vi "set_detectors.vi"(8 "error in (no error)":errorcluster, 11 "DET_BUNCH in":refnum<class "Avantes_bunch.lvclass">) -> (0 "error out":errorcluster, 3 "DET_BUNCH out":refnum<class "Avantes_bunch.lvclass">)   [LabVIEW 2020, in "Avantes_bunch.lvclass"]
uses:
  Avantes_bunch.lvclass
  C:/Dev/TRANCON/Classes/GeneralFunctionality/GeneralFunctionality.lvclass
  GeneralFunctionality/GeneralFunctionality.lvclass/GeneralFunctionality.ctl
  Config/Config.lvclass
  UV-VIS_AVANTES/UV-VIS_AVANTES.lvclass
  C:/Dev/TRANCON/Classes/Detector/Detector.lvclass
  Config/Config.lvclass/Config.ctl
  UV-VIS_AVANTES/UV-VIS_AVANTES.lvclass/UV-VIS_AVANTES.ctl
  Avantes_bunch.lvclass/Avantes_bunch.ctl
  <userlib>/_OpenG.lib/dictionary/dictionary.llb/Dictionary Create__ogtk.vi
  <userlib>/_OpenG.lib/dictionary/dictionary.llb/Dictionary Update__ogtk.vi
  <userlib>/_OpenG.lib/dictionary/dictionary.llb/Dictionary Update (by scalar value)__ogtk.vi
  <userlib>/_OpenG.lib/dictionary/dictionary.llb/Dictionary Get Value__ogtk.vi
  GeneralFunctionality/GeneralFunctionality.lvclass
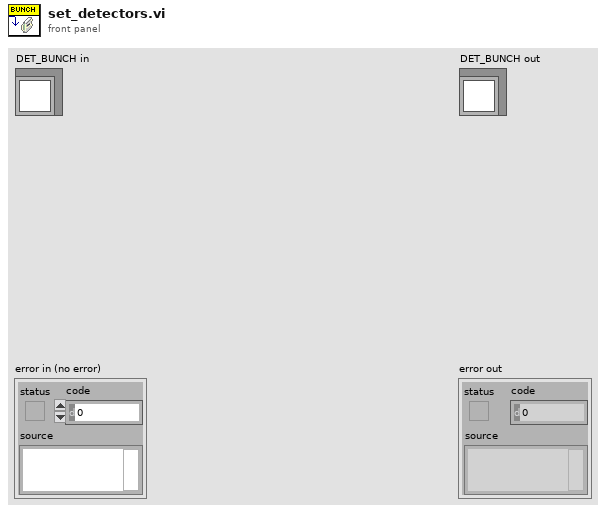
[diagram p1: front panel]
types:
  T1 = typedef "Rendezvous RefNum" = refnum<k1>
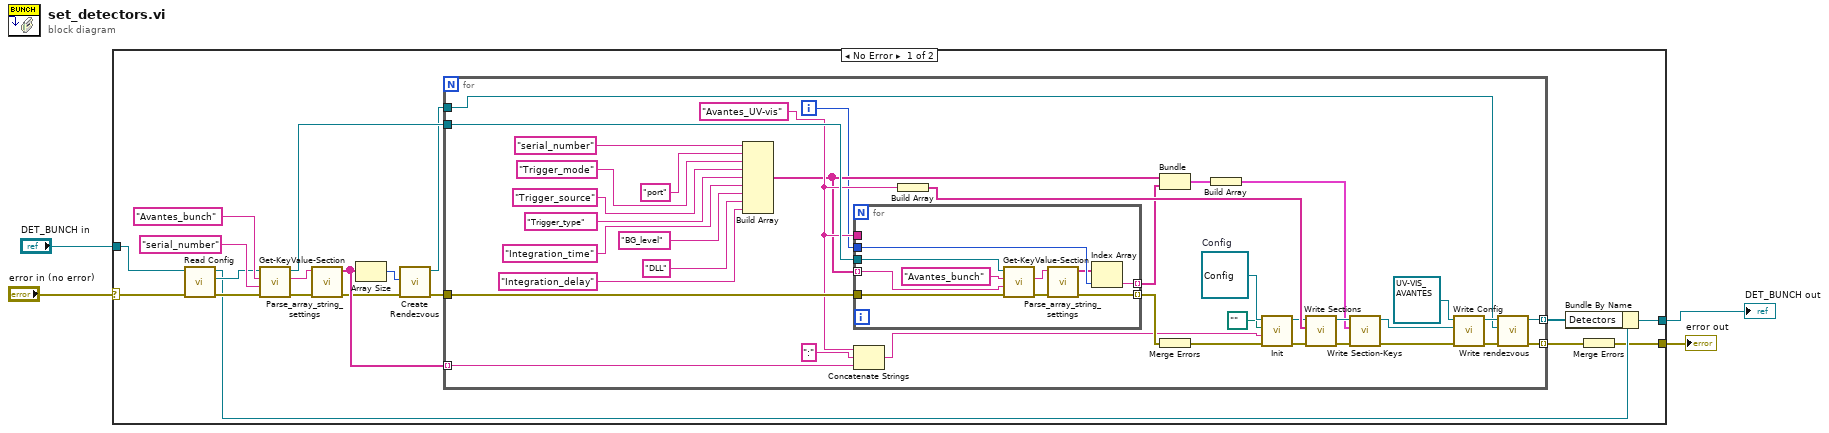
[diagram p0: block diagram]
diagram:
  n1 = case shown="No Error" "error in (no error)" {
    selector: "error in (no error)" -> [w15 w72]
    tunnel: [w11 w72] -> w3
    tunnel: [w10 w71] -> w1
    tunnel: "DET_BUNCH in" -> [w18 w71]
    frame No Error {
      n2 = call "Read Config.vi"("error in (no error)"=w15, "GeneralFunctionality en entrée"=w18) -> ("error out"=w16:errorcluster, "Config.lvclass"=w17:refnum<class "Config.lvclass">, "GeneralFunctionality en sortie"=w14:refnum<class "Avantes_bunch.lvclass">)  [unwired: 7 in]
      n3 = call-dynamic "Get-KeyValue-Section.vi"("error in (no error)"=w16, "Key"="serial_number", "Section"="Avantes_bunch", "Config in"=w17) -> ("error out"=w22:errorcluster, "Value"=w21:string, "Config out"=w23:refnum<class "Config.lvclass">)  [unwired: 5 in]
      n4 = call "Parse_array_string_settings.vi"("error in (no error)"=w22, "Value"=w21) -> ("error out"=w7:errorcluster, "Output"=w9:string[])  [unwired: 8 in]
      n5 = Array Size(array=w9) -> (size(s)=w8:i32)
      n6 = call <vilib>:"Create Rendezvous.vi"("error in (no error)"=w7, "size (2)"=w8) -> ("error out"=w6:errorcluster, "rendezvous"=w5:T1)  [unwired: 3 in, 1 out]
      n7 = for {
        tunnel: w9 -> [w46] mode=indexing
        tunnel: w6 -> [w52]
        tunnel: [w25] -> w12 mode=indexing
        tunnel: w23 -> [w55]
        tunnel: [w26] -> w13 mode=indexing
        tunnel: w5 -> [w24]
        i -> [w34]
        w42 = "Avantes_UV-vis" ("Section")
        w50 = refnum<class "Config.lvclass"> refnum  # Config
        n8 = Build Array("serial_number" ("Key"), "port" ("Key"), "Trigger_mode" ("element"), "Trigger_source" ("element"), "Trigger_type" ("element"), "Integration_time" ("element"), "BG_level" ("element"), "DLL" ("element"), "Integration_delay" ("element")) -> (w40:string[])
        n9 = for {
          tunnel: w55 -> [w70]
          tunnel: w40 -> [w69] mode=indexing
          tunnel: w42 -> [_]
          tunnel: [w64] -> w41 mode=indexing
          tunnel: [w63] -> w51 mode=indexing
          tunnel: w52 -> [w68]
          tunnel: w34 -> [w65]
          n10 = call-dynamic "Get-KeyValue-Section.vi"("error in (no error)"=w68, "Key"=w69, "Section"="Avantes_bunch", "Config in"=w70) -> ("error out"=w62:errorcluster, "Value"=w66:string)  [unwired: 5 in, 1 out]
          n11 = call "Parse_array_string_settings.vi"("error in (no error)"=w62, "Value"=w66) -> ("error out"=w63:errorcluster, "Output"=w61:string[])  [unwired: 8 in]
          n12 = Index Array(array=w61, index=w65) -> (element=w64:string)
        }
        n13 = Concatenate Strings(w42, ":" ("string"), w46) -> (w44:string)
        n14 = Build Array(w42) -> (w59:string[])
        n15 = Bundle(w40, w41) -> (w54:cluster{string[], string[]})  [unwired: 1 in]
        n16 = Merge Errors(w51) -> (w49:errorcluster)
        n17 = Build Array(w54) -> (w33:cluster{string[], string[]}[])
        n18 = call "Init.vi"("error in"=w49, "Name"=w44, "Path"=path "", "Config in"=w50) -> ("error out"=w47:errorcluster, "Config out"=w48:refnum<class "Config.lvclass">)  [unwired: 6 in]
        n19 = call "Write Sections.vi"("error in (no error)"=w47, "Sections"=w59, "Config in"=w48) -> ("error out"=w53:errorcluster, "Config out"=w56:refnum<class "Config.lvclass">)  [unwired: 7 in]
        n20 = call "Write Section-Keys.vi"("error in (no error)"=w53, "Section-Keys"=w33, "Config in"=w56) -> ("error out"=w31:errorcluster, "Config out"=w32:refnum<class "Config.lvclass">)  [unwired: 7 in]
        n21 = call "Write Config.vi"("error in (no error)"=w31, "Config.lvclass"=w32, "GeneralFunctionality en entrée"=refnum<class "UV-VIS_AVANTES.lvclass"> refnum ("UV-VIS_AVANTES.lvclass")) -> ("error out"=w28:errorcluster, "GeneralFunctionality en sortie"=w27:refnum<class "UV-VIS_AVANTES.lvclass">)  [unwired: 7 in]
        n22 = call "Write rendezvous.vi"("error in (no error)"=w28, "rendezvous"=w24, "UV-VIS_AVANTES in"=w27) -> ("error out"=w25:errorcluster, "UV-VIS_AVANTES out"=w26:refnum<class "UV-VIS_AVANTES.lvclass">)  [unwired: 7 in]
      }
      n23 = Bundle By Name(cluster=w14, "Detectors"=w13) -> (w10:refnum<class "Avantes_bunch.lvclass">)
      n24 = Merge Errors(w12) -> (w11:errorcluster)
    }
    frame Error {
    }
  }
  "error out" <- w3
  "DET_BUNCH out" <- w1
